vi "Run Process Queue.vi"(6 "Currrent Step":string, 8 "Queue Reactor X":refnum<vi>, 9 "Current Cycle Reactor X":refnum<vi>, 10 "Start Time Reactor X":refnum<vi>, 11 "GUID X":refnum<vi>) -> ()   [LabVIEW 2022 SP3]
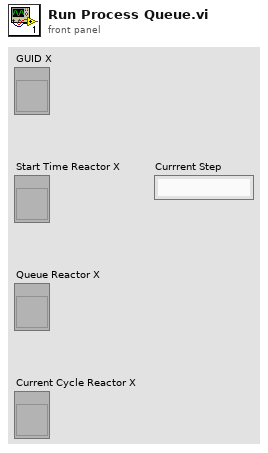
[diagram p1: front panel]
types:
  T1 = cluster{"TimeElapsed":string, "CurrentCycle":string, "CurrentStep":string, "GUID":string}
  T2 = cluster{"type":string, "meta":string, "payload":string}
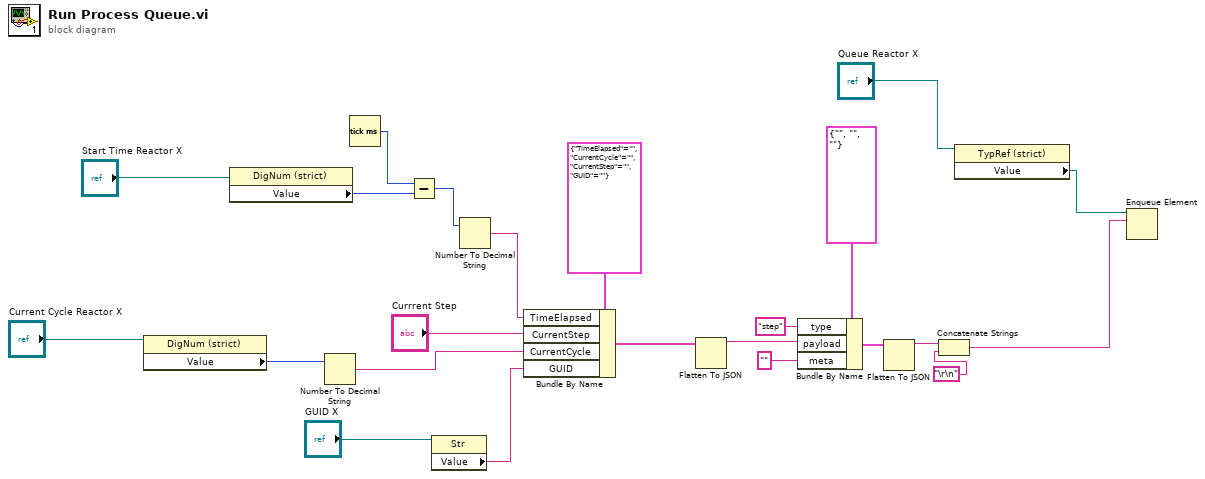
[diagram p0: block diagram]
diagram:
  n1 = property class="DigNum (strict)"(reference="Current Cycle Reactor X") -> ("Value"=w6:i32)  [unwired: 1 in, 2 out]
  n2 = property class="DigNum (strict)"(reference="Start Time Reactor X") -> ("Value"=w17:i32)  [unwired: 1 in, 2 out]
  n3 = Number To Decimal String(number=w6) -> (decimal integer string=w4:string)  [unwired: 1 in]
  n4 = Tick Count (ms)() -> (millisecond timer value=w16:u32)
  n5 = Subtract(x=w16, y=w17) -> (x-y=w20:u32)
  n6 = property class="Str"(reference="GUID X") -> ("Value"=w23:string)  [unwired: 1 in, 2 out]
  n7 = Number To Decimal String(number=w20) -> (decimal integer string=w21:string)  [unwired: 1 in]
  n8 = Bundle By Name(cluster=T1 {"TimeElapsed"="", "CurrentCycle"="", "CurrentStep"="", "GUID"=""} ("input cluster"), "TimeElapsed"=w21, "CurrentStep"="Currrent Step", "CurrentCycle"=w4, "GUID"=w23) -> (w18:T1)
  n9 = Flatten To JSON(anything=w18) -> (JSON string=w19:string)  [unwired: 2 in, 1 out]
  n10 = Bundle By Name(cluster=T2 {"type"="", "meta"="", "payload"=""} ("input cluster"), "type"="step", "payload"=w19, "meta"="") -> (w10:T2)
  n11 = Flatten To JSON(anything=w10) -> (JSON string=w9:string)  [unwired: 2 in, 1 out]
  n12 = Concatenate Strings(w9, "\r\n") -> (w2:string)
  n13 = property class="TypRef (strict)"(reference="Queue Reactor X") -> ("Value"=w3:refnum<queue>)  [unwired: 1 in, 2 out]
  n14 = Enqueue Element(queue=w3, element=w2) -> ()  [unwired: 2 in, 3 out]
